vi "Get next acquisition state.vi"(10 "Acquisition order":T2(ring), 11 "Acquisition cluster in":T1={"Save path"=path "D:/DATA_2018", "t frame"=0, "bookmark #"=0, "Z-current"=0, "Channel"=0, "total t frames"=0, "Total bookmarks"=0, "Total z steps"=0, "Total channels"=0, "Gain 1"=100, "Gain 2"=100, "Gain 3"=100, "Gain 4"=100, "Exposure 1"=100.0, "Exposure 2"=100.0, "Exposure 3"=100.0, "Exposure 4"=100.0, "Channel 1"="Red", "Channel 2"="None", "Channel 3"="None", "Channel 4"="None", "Bookmarks?"=FALSE, "Acquisition order"=enum."C-T-Z-B", "t-delay"=0.0, "z-step"=1.0, "Total Images"=1, "Start position"=[], "Piezo radio"=enum."Piezo off", "Piezo Step X"=20.0, "Piezo Step Y"=20.0, "Piezo Step Z"=20.0, "Piezo X current"=0.0, "Piezo Y current"=0.0, "Piezo Z current"=0.0, "LED illumination"=TRUE, "Piezo Amp X"=0.0, "Piezo Amp Y"=0.0, "Piezo Amp Z"=0.0}) -> (0 "Next state":T3 caption="States", 3 "Acquisition cluster out":T1={"Save path"=path "D:/DATA_2018", "t frame"=0, "bookmark #"=0, "Z-current"=0, "Channel"=0, "total t frames"=0, "Total bookmarks"=0, "Total z steps"=0, "Total channels"=0, "Gain 1"=100, "Gain 2"=100, "Gain 3"=100, "Gain 4"=100, "Exposure 1"=100.0, "Exposure 2"=100.0, "Exposure 3"=100.0, "Exposure 4"=100.0, "Channel 1"="Red", "Channel 2"="None", "Channel 3"="None", "Channel 4"="None", "Bookmarks?"=FALSE, "Acquisition order"=enum."C-T-Z-B", "t-delay"=0.0, "z-step"=1.0, "Total Images"=1, "Start position"=[], "Piezo radio"=enum."Piezo off", "Piezo Step X"=20.0, "Piezo Step Y"=20.0, "Piezo Step Z"=20.0, "Piezo X current"=0.0, "Piezo Y current"=0.0, "Piezo Z current"=0.0, "LED illumination"=TRUE, "Piezo Amp X"=0.0, "Piezo Amp Y"=0.0, "Piezo Amp Z"=0.0})   [LabVIEW 2017]
uses:
  <instrlib>/TLDC4100/TLDC4100.llb/z_StateMachineVorlage.ctl
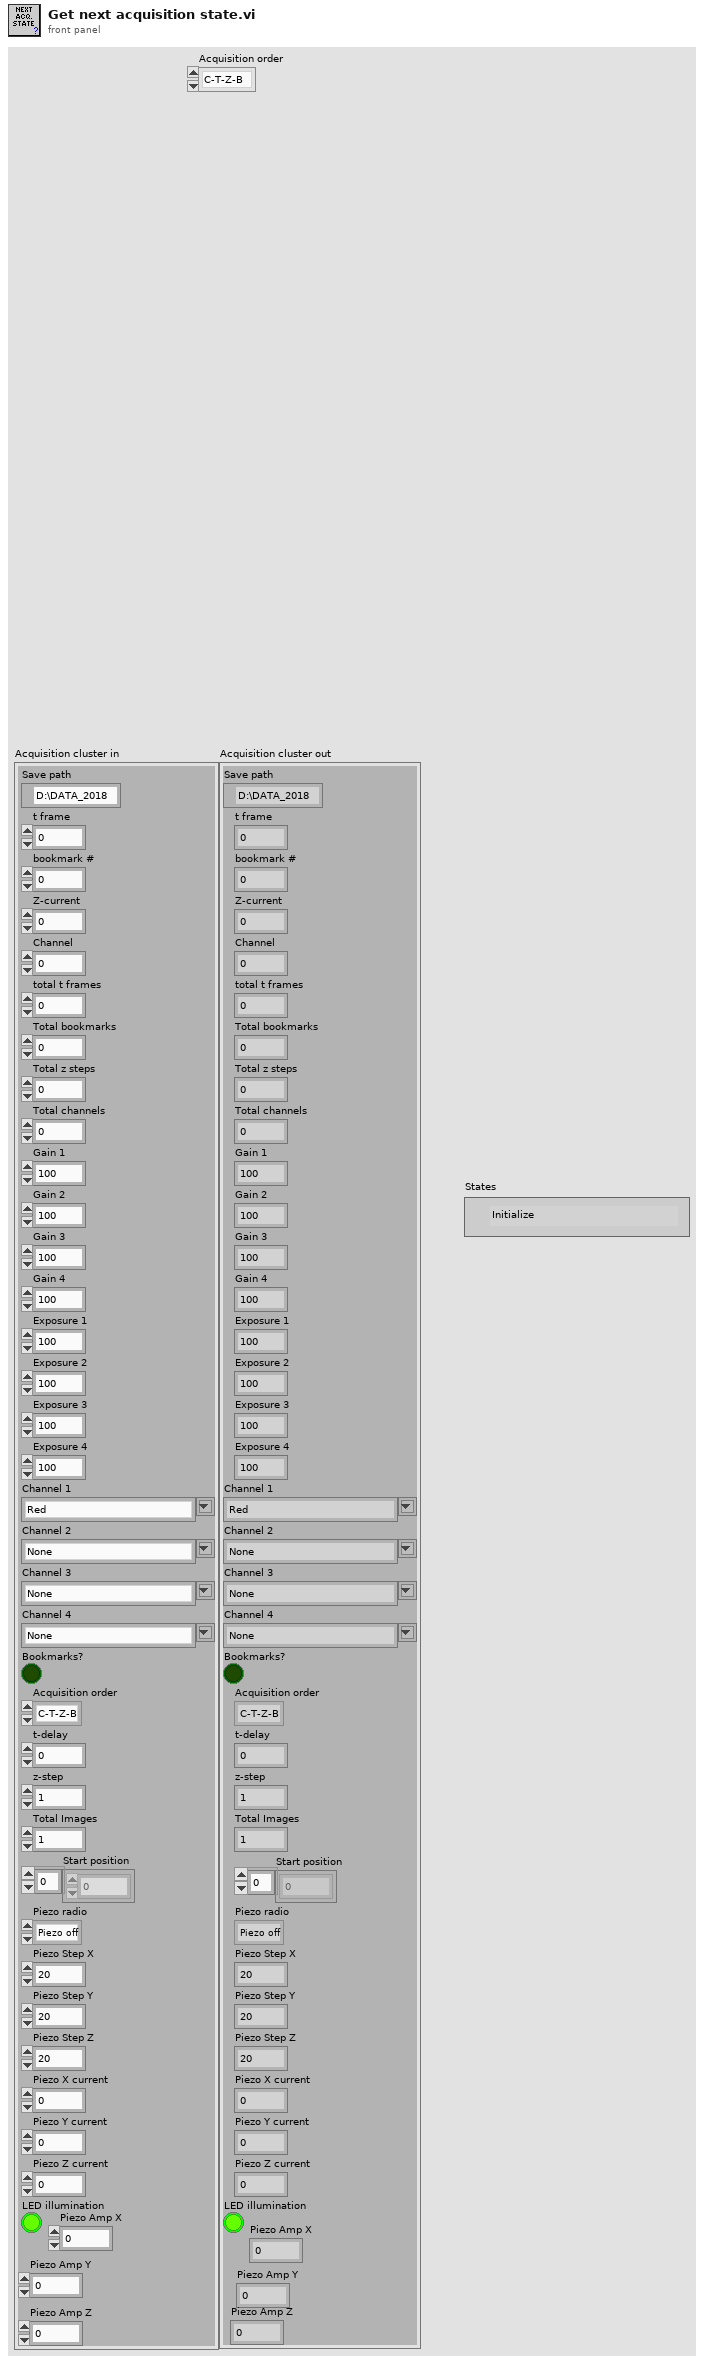
[diagram p1: front panel]
types:
  T1 = cluster{"Save path":path, "t frame":i32, "bookmark #":i32, "Z-current":i32, "Channel":i32, "total t frames":i32, "Total bookmarks":i32, "Total z steps":i32, "Total channels":i32, "Gain 1":i32, "Gain 2":i32, "Gain 3":i32, "Gain 4":i32, "Exposure 1":dbl, "Exposure 2":dbl, "Exposure 3":dbl, "Exposure 4":dbl, "Channel 1":string, "Channel 2":string, "Channel 3":string, "Channel 4":string, "Bookmarks?":bool, "Acquisition order":enum16{"C-T-Z-B", "C-T-B-Z", "C-Z-T-B", "C-Z-B-T", "C-B-T-Z", "C-B-Z-T", "T-C-Z-B", "T-C-B-Z", "T-Z-C-B", "T-Z-B-C", "T-B-C-Z", "T-B-Z-C", "Z-C-T-B", "Z-C-B-T", "Z-T-C-B", "Z-T-B-C", "Z-B-C-T", "Z-B-T-C", "B-C-T-Z", "B-C-Z-T", "B-Z-C-T", "B-Z-T-C", "B-T-C-Z", "B-T-Z-C"}, "t-delay":dbl, "z-step":dbl, "Total Images":i32, "Start position":dbl[], "Piezo radio":enum32{"Piezo off", "Piezo wiggle", "Piezo step"}, "Piezo Step X":dbl, "Piezo Step Y":dbl, "Piezo Step Z":dbl, "Piezo X current":dbl, "Piezo Y current":dbl, "Piezo Z current":dbl, "LED illumination":bool, "Piezo Amp X":dbl, "Piezo Amp Y":dbl, "Piezo Amp Z":dbl}
  T2 = enum16{"C-T-Z-B", "C-T-B-Z", "C-Z-T-B", "C-Z-B-T", "C-B-T-Z", "C-B-Z-T", "T-C-Z-B", "T-C-B-Z", "T-Z-C-B", "T-Z-B-C", "T-B-C-Z", "T-B-Z-C", "Z-C-T-B", "Z-C-B-T", "Z-T-C-B", "Z-T-B-C", "Z-B-C-T", "Z-B-T-C", "B-C-T-Z", "B-C-Z-T", "B-Z-C-T", "B-Z-T-C", "B-T-C-Z", "B-T-Z-C"}
  T3 = typedef "z_StateMachineVorlage.ctl" = enum16{"Initialize", "1", "2", "3", "4", "5", "6", "7", "8", "9", "10", "11", "12", "13", "14", "15", "20", "25", "30", "35", "40", "45", "50", "55", "59", "60", "65", "70", "75", "76", "77", "78", "79", "80", "85", "90", "91", "92", "93", "94", "95", "96", "97", "98", "99", "100", "105", "110", "120", "130", "140", "150", "160", "170", "180", "190", "200", "201", "202", "203", "205", "210", "215", "220", "230", "240", "245", "250", "255", "260", "270", "280", "290", "300", "310", "313", "315", "318", "320", "330", "340", "350", "360", "370", "380", "390", "400", "410", "420", "430", "440", "450", "460", "470", "480", "490", "500", "501", "502", "503", "504", "505", "506", "507", "510", "511", "512", "513", "514", "520", "523", "525", "528", "530", "540", "550", "560", "570", "580", "590", "591", "592", "593", "600", "601", "602", "605", "610", "620", "630", "640", "650", "660", "670", "680", "690", "700", "710", "720", "730", "740", "750", "760", "770", "780", "790", "800", "810", "820", "830", "840", "850", "860", "870", "880", "890", "900", "910", "920", "930", "940", "950", "960", "970", "980", "990", "1000", "1010", "1020", "1030", "1040", "1050", "1060", "1070", "1080", "1090", "1100", "1110", "1120", "1130", "1140", "1150", "1160", "1170", "1180", "1190", "1200", "1210", "1220", "1230", "1240", "1250", "1260", "1270", "1280", "1290", "1300", "1310", "1320", "1330", "1340", "1350", "1360", "1370", "1380", "1390", "1400", "1410", "1420", "1430", "1440", "1450", "1460", "1470", "1480", "1490", "1500", "Fehler I", "Fehler II", "Fehler III", "Fehler IV", "Fehler V", "Fehler VI", "Fehler VII", "Fehler VIII", "Fehler IX", "Fehler X", "Stop"}
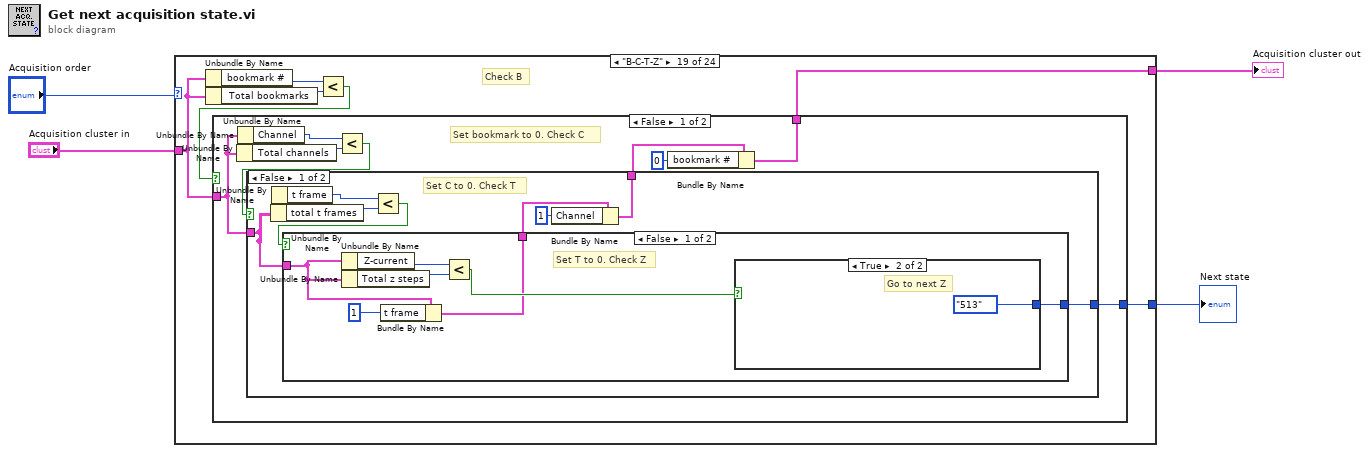
[diagram p0: block diagram]
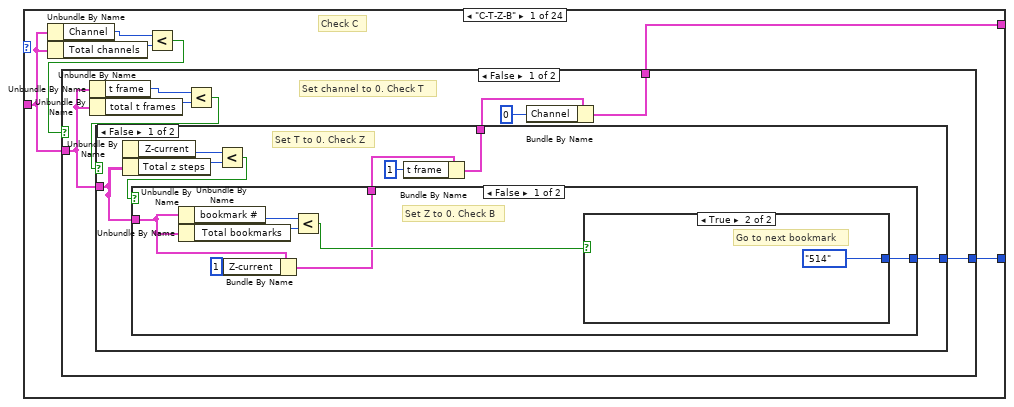
[diagram p2: hidden frame]
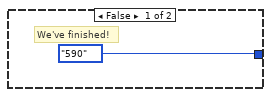
[diagram p3: hidden frame]
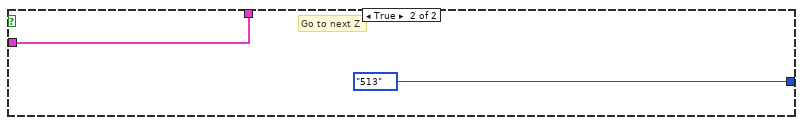
[diagram p4: hidden frame]
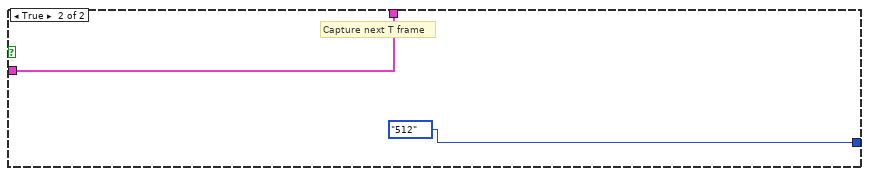
[diagram p5: hidden frame]
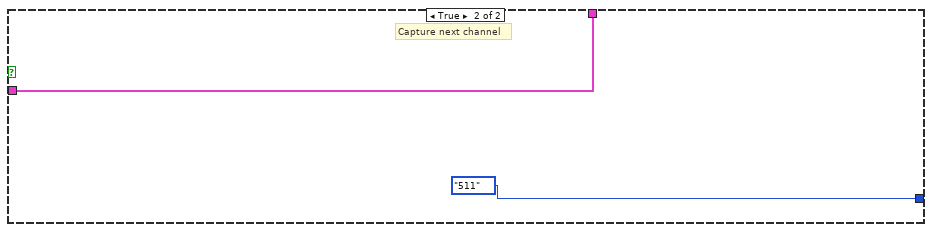
[diagram p6: hidden frame]
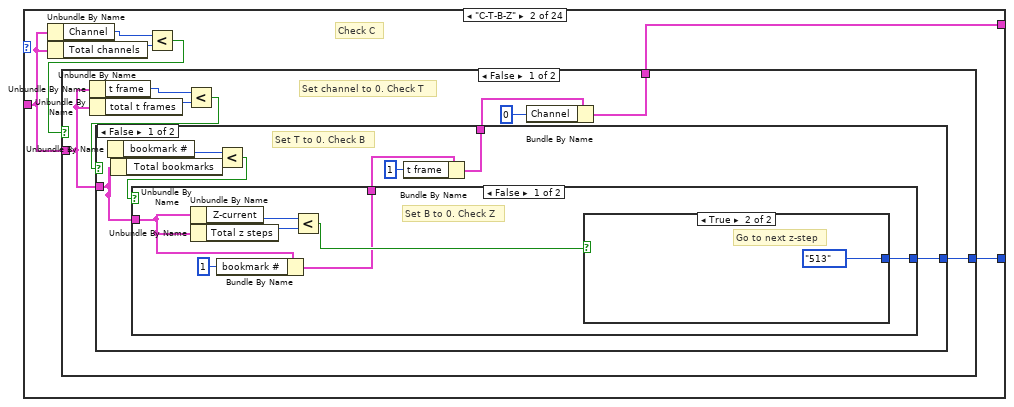
[diagram p7: hidden frame]
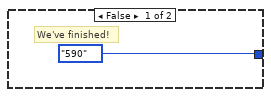
[diagram p8: hidden frame]
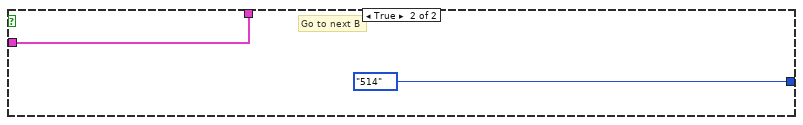
[diagram p9: hidden frame]
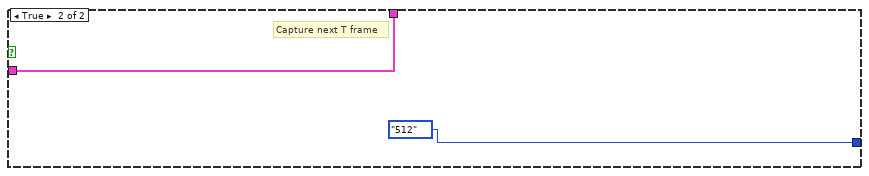
[diagram p10: hidden frame]
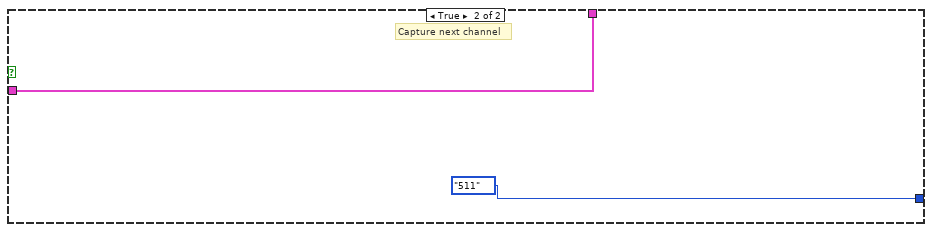
[diagram p11: hidden frame]
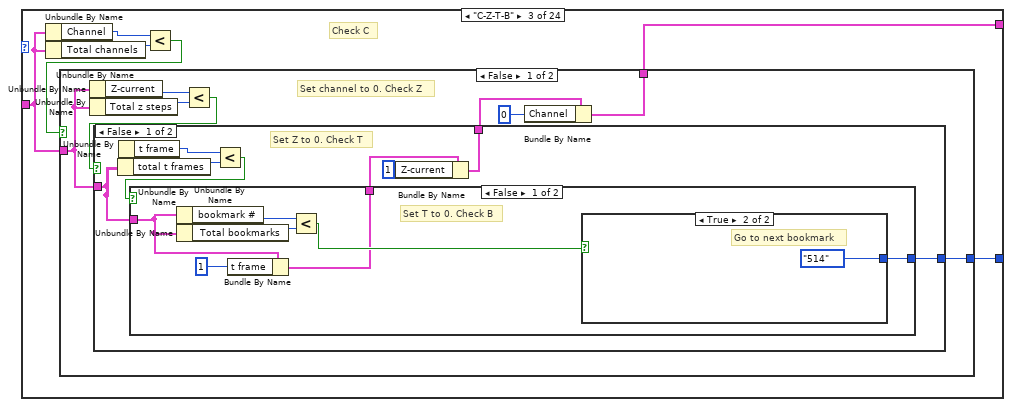
[diagram p12: hidden frame]
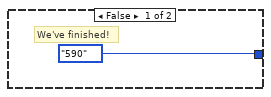
[diagram p13: hidden frame]
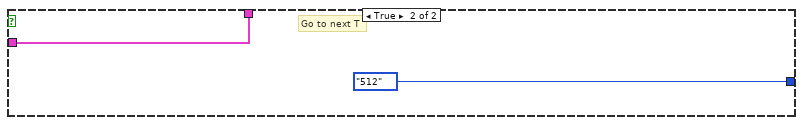
[diagram p14: hidden frame]
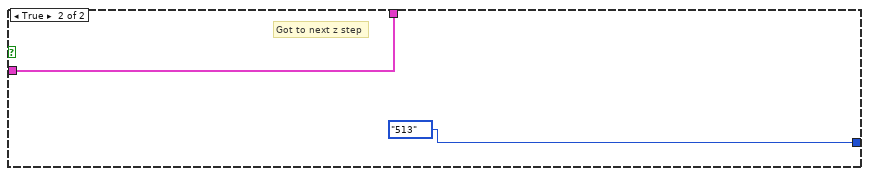
[diagram p15: hidden frame]
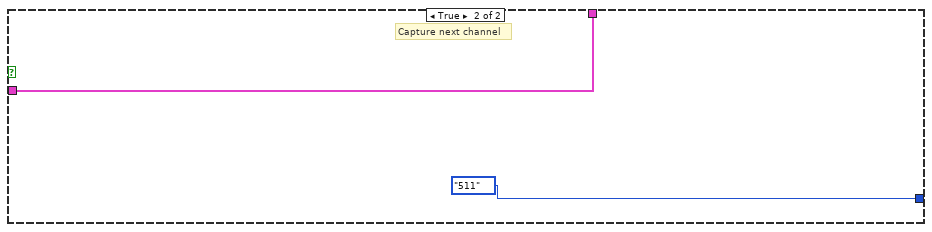
[diagram p16: hidden frame]
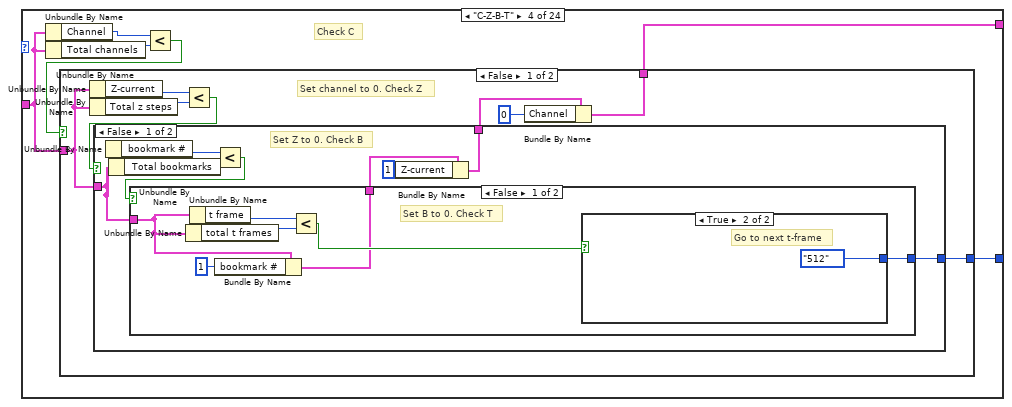
[diagram p17: hidden frame]
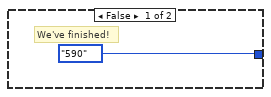
[diagram p18: hidden frame]
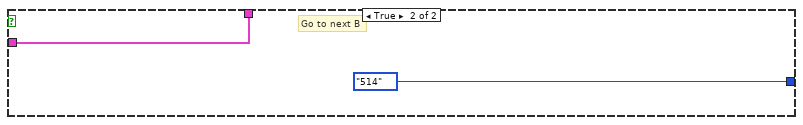
[diagram p19: hidden frame]
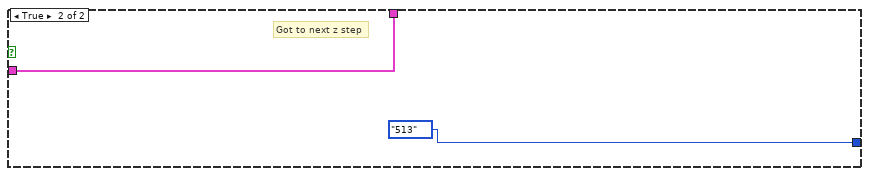
[diagram p20: hidden frame]
diagram:
  n1 = case shown="\"B-C-T-Z\"" "Acquisition order" {
    tunnel: "Acquisition cluster in" -> [w7 w44 w81 w118 w155 w192 w229 w266 w303 w340 w377 w414 w451 w488 w525 w562 w599 w636 w673 w710 w747 w784 w821 w858]
    tunnel: [w6 w43 w80 w117 w154 w191 w228 w265 w302 w339 w376 w413 w450 w487 w524 w561 w598 w635 w672 w709 w746 w783 w820 w857] -> w3
    tunnel: [w5 w42 w79 w116 w153 w190 w227 w264 w301 w338 w375 w412 w449 w486 w523 w560 w597 w634 w671 w708 w745 w782 w819 w856] -> w1
    frame "C-T-Z-B" {
      # "Check C"
      n2 = Unbundle By Name(w7) -> ("Channel"=w10:i32)
      n3 = Unbundle By Name(w7) -> ("Total channels"=w9:i32)
      n4 = Less?(x=w10, y=w9) -> (x < y?=w8:bool)
      n5 = case shown="False" w8 {
        tunnel: w7 -> [w14 w40]
        tunnel: [w15 z_StateMachineVorlage."511" ("States")] -> w6
        tunnel: [w11 w40] -> w5
        frame False {
          # "Set channel to 0. Check T"
          n6 = Unbundle By Name(w14) -> ("t frame"=w17:i32)
          n7 = Unbundle By Name(w14) -> ("total t frames"=w18:i32)
          n8 = Less?(x=w17, y=w18) -> (x < y?=w16:bool)
          n9 = case shown="False" w16 {
            tunnel: [w23 z_StateMachineVorlage."512" ("States")] -> w15
            tunnel: w14 -> [w22 w38]
            tunnel: [w19 w38] -> w12
            frame False {
              # "Set T to 0. Check Z"
              n10 = Unbundle By Name(w22) -> ("Z-current"=w26:i32)
              n11 = Unbundle By Name(w22) -> ("Total z steps"=w25:i32)
              n12 = Less?(x=w26, y=w25) -> (x < y?=w24:bool)
              n13 = case shown="False" w24 {
                tunnel: w22 -> [w29 w36]
                tunnel: [w30 z_StateMachineVorlage."513" ("States")] -> w23
                tunnel: [w27 w36] -> w20
                frame False {
                  # "Set Z to 0. Check B"
                  n14 = Unbundle By Name(w29) -> ("bookmark #"=w32:i32)
                  n15 = Unbundle By Name(w29) -> ("Total bookmarks"=w33:i32)
                  n16 = Bundle By Name(cluster=w29, "Z-current"=1 ("Z-step")) -> (w27:T1)
                  n17 = Less?(x=w32, y=w33) -> (x < y?=w31:bool)
                  n18 = case shown="True" w31 {
                    tunnel: [z_StateMachineVorlage."590" ("States") z_StateMachineVorlage."514" ("States")] -> w30
                    frame False {
                      # "We've finished!"
                    }
                    frame True {
                      # "Go to next bookmark"
                    }
                  }
                }
                frame True {
                  # "Go to next Z"
                }
              }
              n19 = Bundle By Name(cluster=w20, "t frame"=1 ("Z-step")) -> (w19:T1)
            }
            frame True {
              # "Capture next T frame"
            }
          }
          n20 = Bundle By Name(cluster=w12, "Channel"=0 ("Z-step")) -> (w11:T1)
        }
        frame True {
          # "Capture next channel"
        }
      }
    }
    frame "C-T-B-Z" {
      # "Check C"
      n21 = Unbundle By Name(w44) -> ("Channel"=w47:i32)
      n22 = Unbundle By Name(w44) -> ("Total channels"=w46:i32)
      n23 = Less?(x=w47, y=w46) -> (x < y?=w45:bool)
      n24 = case shown="False" w45 {
        tunnel: w44 -> [w51 w77]
        tunnel: [w52 z_StateMachineVorlage."511" ("States")] -> w43
        tunnel: [w48 w77] -> w42
        frame False {
          # "Set channel to 0. Check T"
          n25 = Unbundle By Name(w51) -> ("t frame"=w54:i32)
          n26 = Unbundle By Name(w51) -> ("total t frames"=w55:i32)
          n27 = Less?(x=w54, y=w55) -> (x < y?=w53:bool)
          n28 = case shown="False" w53 {
            tunnel: [w60 z_StateMachineVorlage."512" ("States")] -> w52
            tunnel: w51 -> [w59 w75]
            tunnel: [w56 w75] -> w49
            frame False {
              # "Set T to 0. Check B"
              n29 = Unbundle By Name(w59) -> ("bookmark #"=w63:i32)
              n30 = Unbundle By Name(w59) -> ("Total bookmarks"=w62:i32)
              n31 = Less?(x=w63, y=w62) -> (x < y?=w61:bool)
              n32 = case shown="False" w61 {
                tunnel: w59 -> [w66 w73]
                tunnel: [w67 z_StateMachineVorlage."514" ("States")] -> w60
                tunnel: [w64 w73] -> w57
                frame False {
                  # "Set B to 0. Check Z"
                  n33 = Unbundle By Name(w66) -> ("Z-current"=w69:i32)
                  n34 = Unbundle By Name(w66) -> ("Total z steps"=w70:i32)
                  n35 = Bundle By Name(cluster=w66, "bookmark #"=1 ("Z-step")) -> (w64:T1)
                  n36 = Less?(x=w69, y=w70) -> (x < y?=w68:bool)
                  n37 = case shown="True" w68 {
                    tunnel: [z_StateMachineVorlage."590" ("States") z_StateMachineVorlage."513" ("States")] -> w67
                    frame False {
                      # "We've finished!"
                    }
                    frame True {
                      # "Go to next z-step"
                    }
                  }
                }
                frame True {
                  # "Go to next B"
                }
              }
              n38 = Bundle By Name(cluster=w57, "t frame"=1 ("Z-step")) -> (w56:T1)
            }
            frame True {
              # "Capture next T frame"
            }
          }
          n39 = Bundle By Name(cluster=w49, "Channel"=0 ("Z-step")) -> (w48:T1)
        }
        frame True {
          # "Capture next channel"
        }
      }
    }
    frame "C-Z-T-B" {
      # "Check C"
      n40 = Unbundle By Name(w81) -> ("Channel"=w84:i32)
      n41 = Unbundle By Name(w81) -> ("Total channels"=w83:i32)
      n42 = Less?(x=w84, y=w83) -> (x < y?=w82:bool)
      n43 = case shown="False" w82 {
        tunnel: w81 -> [w88 w114]
        tunnel: [w89 z_StateMachineVorlage."511" ("States")] -> w80
        tunnel: [w85 w114] -> w79
        frame False {
          # "Set channel to 0. Check Z"
          n44 = Unbundle By Name(w88) -> ("Z-current"=w91:i32)
          n45 = Unbundle By Name(w88) -> ("Total z steps"=w92:i32)
          n46 = Less?(x=w91, y=w92) -> (x < y?=w90:bool)
          n47 = case shown="False" w90 {
            tunnel: [w97 z_StateMachineVorlage."513" ("States")] -> w89
            tunnel: w88 -> [w96 w112]
            tunnel: [w93 w112] -> w86
            frame False {
              # "Set Z to 0. Check T"
              n48 = Unbundle By Name(w96) -> ("total t frames"=w99:i32)
              n49 = Unbundle By Name(w96) -> ("t frame"=w100:i32)
              n50 = Less?(x=w100, y=w99) -> (x < y?=w98:bool)
              n51 = case shown="False" w98 {
                tunnel: w96 -> [w103 w110]
                tunnel: [w104 z_StateMachineVorlage."512" ("States")] -> w97
                tunnel: [w101 w110] -> w94
                frame False {
                  # "Set T to 0. Check B"
                  n52 = Unbundle By Name(w103) -> ("bookmark #"=w106:i32)
                  n53 = Unbundle By Name(w103) -> ("Total bookmarks"=w107:i32)
                  n54 = Bundle By Name(cluster=w103, "t frame"=1 ("Z-step")) -> (w101:T1)
                  n55 = Less?(x=w106, y=w107) -> (x < y?=w105:bool)
                  n56 = case shown="True" w105 {
                    tunnel: [z_StateMachineVorlage."590" ("States") z_StateMachineVorlage."514" ("States")] -> w104
                    frame False {
                      # "We've finished!"
                    }
                    frame True {
                      # "Go to next bookmark"
                    }
                  }
                }
                frame True {
                  # "Go to next T"
                }
              }
              n57 = Bundle By Name(cluster=w94, "Z-current"=1 ("Z-step")) -> (w93:T1)
            }
            frame True {
              # "Got to next z step"
            }
          }
          n58 = Bundle By Name(cluster=w86, "Channel"=0 ("Z-step")) -> (w85:T1)
        }
        frame True {
          # "Capture next channel"
        }
      }
    }
    frame "C-Z-B-T" {
      # "Check C"
      n59 = Unbundle By Name(w118) -> ("Channel"=w121:i32)
      n60 = Unbundle By Name(w118) -> ("Total channels"=w120:i32)
      n61 = Less?(x=w121, y=w120) -> (x < y?=w119:bool)
      n62 = case shown="False" w119 {
        tunnel: w118 -> [w125 w151]
        tunnel: [w126 z_StateMachineVorlage."511" ("States")] -> w117
        tunnel: [w122 w151] -> w116
        frame False {
          # "Set channel to 0. Check Z"
          n63 = Unbundle By Name(w125) -> ("Z-current"=w128:i32)
          n64 = Unbundle By Name(w125) -> ("Total z steps"=w129:i32)
          n65 = Less?(x=w128, y=w129) -> (x < y?=w127:bool)
          n66 = case shown="False" w127 {
            tunnel: [w134 z_StateMachineVorlage."513" ("States")] -> w126
            tunnel: w125 -> [w133 w149]
            tunnel: [w130 w149] -> w123
            frame False {
              # "Set Z to 0. Check B"
              n67 = Unbundle By Name(w133) -> ("bookmark #"=w137:i32)
              n68 = Unbundle By Name(w133) -> ("Total bookmarks"=w136:i32)
              n69 = Less?(x=w137, y=w136) -> (x < y?=w135:bool)
              n70 = case shown="False" w135 {
                tunnel: w133 -> [w140 w147]
                tunnel: [w141 z_StateMachineVorlage."514" ("States")] -> w134
                tunnel: [w138 w147] -> w131
                frame False {
                  # "Set B to 0. Check T"
                  n71 = Unbundle By Name(w140) -> ("total t frames"=w144:i32)
                  n72 = Unbundle By Name(w140) -> ("t frame"=w143:i32)
                  n73 = Bundle By Name(cluster=w140, "bookmark #"=1 ("Z-step")) -> (w138:T1)
                  n74 = Less?(x=w143, y=w144) -> (x < y?=w142:bool)
                  n75 = case shown="True" w142 {
                    tunnel: [z_StateMachineVorlage."590" ("States") z_StateMachineVorlage."512" ("States")] -> w141
                    frame False {
                      # "We've finished!"
                    }
                    frame True {
                      # "Go to next t-frame"
                    }
                  }
                }
                frame True {
                  # "Go to next B"
                }
              }
              n76 = Bundle By Name(cluster=w131, "Z-current"=1 ("Z-step")) -> (w130:T1)
            }
            frame True {
              # "Got to next z step"
            }
          }
          n77 = Bundle By Name(cluster=w123, "Channel"=0 ("Z-step")) -> (w122:T1)
        }
        frame True {
          # "Capture next channel"
        }
      }
    }
    frame "C-B-T-Z" {
      # "Check C"
      n78 = Unbundle By Name(w155) -> ("Channel"=w158:i32)
      n79 = Unbundle By Name(w155) -> ("Total channels"=w157:i32)
      n80 = Less?(x=w158, y=w157) -> (x < y?=w156:bool)
      n81 = case shown="False" w156 {
        tunnel: w155 -> [w162 w188]
        tunnel: [w163 z_StateMachineVorlage."511" ("States")] -> w154
        tunnel: [w159 w188] -> w153
        frame False {
          # "Set channel to 0. Check Z"
          n82 = Unbundle By Name(w162) -> ("bookmark #"=w165:i32)
          n83 = Unbundle By Name(w162) -> ("Total bookmarks"=w166:i32)
          n84 = Less?(x=w165, y=w166) -> (x < y?=w164:bool)
          n85 = case shown="False" w164 {
            tunnel: [w171 z_StateMachineVorlage."514" ("States")] -> w163
            tunnel: w162 -> [w170 w186]
            tunnel: [w167 w186] -> w160
            frame False {
              # "Set B to 0. Check T"
              n86 = Unbundle By Name(w170) -> ("total t frames"=w173:i32)
              n87 = Unbundle By Name(w170) -> ("t frame"=w174:i32)
              n88 = Less?(x=w174, y=w173) -> (x < y?=w172:bool)
              n89 = case shown="False" w172 {
                tunnel: w170 -> [w177 w184]
                tunnel: [w178 z_StateMachineVorlage."512" ("States")] -> w171
                tunnel: [w175 w184] -> w168
                frame False {
                  # "Set T to 0. Check Z"
                  n90 = Unbundle By Name(w177) -> ("Z-current"=w180:i32)
                  n91 = Unbundle By Name(w177) -> ("Total z steps"=w181:i32)
                  n92 = Bundle By Name(cluster=w177, "t frame"=1 ("Z-step")) -> (w175:T1)
                  n93 = Less?(x=w180, y=w181) -> (x < y?=w179:bool)
                  n94 = case shown="True" w179 {
                    tunnel: [z_StateMachineVorlage."590" ("States") z_StateMachineVorlage."513" ("States")] -> w178
                    frame False {
                      # "We've finished!"
                    }
                    frame True {
                      # "Go to next z-step"
                    }
                  }
                }
                frame True {
                  # "Go to next T"
                }
              }
              n95 = Bundle By Name(cluster=w168, "bookmark #"=1 ("Z-step")) -> (w167:T1)
            }
            frame True {
              # "Got to next bookmark"
            }
          }
          n96 = Bundle By Name(cluster=w160, "Channel"=0 ("Z-step")) -> (w159:T1)
        }
        frame True {
          # "Capture next channel"
        }
      }
    }
    frame "C-B-Z-T" {
      # "Check C"
      n97 = Unbundle By Name(w192) -> ("Channel"=w195:i32)
      n98 = Unbundle By Name(w192) -> ("Total channels"=w194:i32)
      n99 = Less?(x=w195, y=w194) -> (x < y?=w193:bool)
      n100 = case shown="False" w193 {
        tunnel: w192 -> [w199 w225]
        tunnel: [w200 z_StateMachineVorlage."511" ("States")] -> w191
        tunnel: [w196 w225] -> w190
        frame False {
          # "Set channel to 0. Check Z"
          n101 = Unbundle By Name(w199) -> ("bookmark #"=w202:i32)
          n102 = Unbundle By Name(w199) -> ("Total bookmarks"=w203:i32)
          n103 = Less?(x=w202, y=w203) -> (x < y?=w201:bool)
          n104 = case shown="False" w201 {
            tunnel: [w208 z_StateMachineVorlage."514" ("States")] -> w200
            tunnel: w199 -> [w207 w223]
            tunnel: [w204 w223] -> w197
            frame False {
              # "Set B to 0. Check Z"
              n105 = Unbundle By Name(w207) -> ("Z-current"=w211:i32)
              n106 = Unbundle By Name(w207) -> ("Total z steps"=w210:i32)
              n107 = Less?(x=w211, y=w210) -> (x < y?=w209:bool)
              n108 = case shown="False" w209 {
                tunnel: w207 -> [w214 w221]
                tunnel: [w215 z_StateMachineVorlage."513" ("States")] -> w208
                tunnel: [w212 w221] -> w205
                frame False {
                  # "Set Z to 0. Check T"
                  n109 = Unbundle By Name(w214) -> ("total t frames"=w218:i32)
                  n110 = Unbundle By Name(w214) -> ("t frame"=w217:i32)
                  n111 = Bundle By Name(cluster=w214, "Z-current"=1 ("Z-step")) -> (w212:T1)
                  n112 = Less?(x=w217, y=w218) -> (x < y?=w216:bool)
                  n113 = case shown="True" w216 {
                    tunnel: [z_StateMachineVorlage."590" ("States") z_StateMachineVorlage."512" ("States")] -> w215
                    frame False {
                      # "We've finished!"
                    }
                    frame True {
                      # "Go to next t-frame"
                    }
                  }
                }
                frame True {
                  # "Go to next Z"
                }
              }
              n114 = Bundle By Name(cluster=w205, "bookmark #"=1 ("Z-step")) -> (w204:T1)
            }
            frame True {
              # "Got to next bookmark"
            }
          }
          n115 = Bundle By Name(cluster=w197, "Channel"=0 ("Z-step")) -> (w196:T1)
        }
        frame True {
          # "Capture next channel"
        }
      }
    }
    frame "T-C-Z-B" {
      # "Check T"
      n116 = Unbundle By Name(w229) -> ("t frame"=w232:i32)
      n117 = Unbundle By Name(w229) -> ("total t frames"=w231:i32)
      n118 = Less?(x=w232, y=w231) -> (x < y?=w230:bool)
      n119 = case shown="False" w230 {
        tunnel: w229 -> [w236 w262]
        tunnel: [w237 z_StateMachineVorlage."512" ("States")] -> w228
        tunnel: [w233 w262] -> w227
        frame False {
          # "Set t-frame to 0. Check C"
          n120 = Unbundle By Name(w236) -> ("Channel"=w239:i32)
          n121 = Unbundle By Name(w236) -> ("Total channels"=w240:i32)
          n122 = Less?(x=w239, y=w240) -> (x < y?=w238:bool)
          n123 = case shown="False" w238 {
            tunnel: [w245 z_StateMachineVorlage."511" ("States")] -> w237
            tunnel: w236 -> [w244 w260]
            tunnel: [w241 w260] -> w234
            frame False {
              # "Set C to 0. Check Z"
              n124 = Unbundle By Name(w244) -> ("Z-current"=w248:i32)
              n125 = Unbundle By Name(w244) -> ("Total z steps"=w247:i32)
              n126 = Less?(x=w248, y=w247) -> (x < y?=w246:bool)
              n127 = case shown="False" w246 {
                tunnel: w244 -> [w251 w258]
                tunnel: [w252 z_StateMachineVorlage."513" ("States")] -> w245
                tunnel: [w249 w258] -> w242
                frame False {
                  # "Set Z to 0. Check B"
                  n128 = Unbundle By Name(w251) -> ("bookmark #"=w254:i32)
                  n129 = Unbundle By Name(w251) -> ("Total bookmarks"=w255:i32)
                  n130 = Bundle By Name(cluster=w251, "Z-current"=1 ("Z-step")) -> (w249:T1)
                  n131 = Less?(x=w254, y=w255) -> (x < y?=w253:bool)
                  n132 = case shown="True" w253 {
                    tunnel: [z_StateMachineVorlage."590" ("States") z_StateMachineVorlage."514" ("States")] -> w252
                    frame False {
                      # "We've finished!"
                    }
                    frame True {
                      # "Go to next bookmark"
                    }
                  }
                }
                frame True {
                  # "Go to next Z"
                }
              }
              n133 = Bundle By Name(cluster=w242, "Channel"=1 ("Z-step")) -> (w241:T1)
            }
            frame True {
              # "Capture next channel"
            }
          }
          n134 = Bundle By Name(cluster=w234, "t frame"=0 ("Z-step")) -> (w233:T1)
        }
        frame True {
          # "Capture next t-frame"
        }
      }
    }
    frame "T-C-B-Z" {
      # "Check T"
      n135 = Unbundle By Name(w266) -> ("t frame"=w269:i32)
      n136 = Unbundle By Name(w266) -> ("total t frames"=w268:i32)
      n137 = Less?(x=w269, y=w268) -> (x < y?=w267:bool)
      n138 = case shown="False" w267 {
        tunnel: w266 -> [w271 w299]
        tunnel: [w270 z_StateMachineVorlage."512" ("States")] -> w265
        tunnel: [w274 w299] -> w264
        frame False {
          # "Set t-frame to 0. Check C"
          n139 = Unbundle By Name(w271) -> ("Channel"=w276:i32)
          n140 = Unbundle By Name(w271) -> ("Total channels"=w277:i32)
          n141 = Less?(x=w276, y=w277) -> (x < y?=w272:bool)
          n142 = case shown="False" w272 {
            tunnel: [w282 z_StateMachineVorlage."511" ("States")] -> w270
            tunnel: w271 -> [w281 w297]
            tunnel: [w278 w297] -> w273
            frame False {
              # "Set C to 0. Check B"
              n143 = Unbundle By Name(w281) -> ("bookmark #"=w285:i32)
              n144 = Unbundle By Name(w281) -> ("Total bookmarks"=w284:i32)
              n145 = Less?(x=w285, y=w284) -> (x < y?=w283:bool)
              n146 = case shown="False" w283 {
                tunnel: w281 -> [w288 w295]
                tunnel: [w289 z_StateMachineVorlage."514" ("States")] -> w282
                tunnel: [w286 w295] -> w279
                frame False {
                  # "Set B to 0. Check Z"
                  n147 = Unbundle By Name(w288) -> ("Z-current"=w291:i32)
                  n148 = Unbundle By Name(w288) -> ("Total z steps"=w292:i32)
                  n149 = Bundle By Name(cluster=w288, "bookmark #"=1 ("Z-step")) -> (w286:T1)
                  n150 = Less?(x=w291, y=w292) -> (x < y?=w290:bool)
                  n151 = case shown="True" w290 {
                    tunnel: [z_StateMachineVorlage."590" ("States") z_StateMachineVorlage."513" ("States")] -> w289
                    frame False {
                      # "We've finished!"
                    }
                    frame True {
                      # "Go to next z-step"
                    }
                  }
                }
                frame True {
                  # "Go to next B"
                }
              }
              n152 = Bundle By Name(cluster=w279, "Channel"=1 ("Z-step")) -> (w278:T1)
            }
            frame True {
              # "Capture next channel"
            }
          }
          n153 = Bundle By Name(cluster=w273, "t frame"=0 ("Z-step")) -> (w274:T1)
        }
        frame True {
          # "Capture next t-frame"
        }
      }
    }
    frame "T-Z-C-B" {
      # "Check T"
      n154 = Unbundle By Name(w303) -> ("t frame"=w306:i32)
      n155 = Unbundle By Name(w303) -> ("total t frames"=w305:i32)
      n156 = Less?(x=w306, y=w305) -> (x < y?=w304:bool)
      n157 = case shown="False" w304 {
        tunnel: w303 -> [w308 w336]
        tunnel: [w307 z_StateMachineVorlage."512" ("States")] -> w302
        tunnel: [w311 w336] -> w301
        frame False {
          # "Set t-frame to 0. Check Z"
          n158 = Unbundle By Name(w308) -> ("Z-current"=w313:i32)
          n159 = Unbundle By Name(w308) -> ("Total z steps"=w314:i32)
          n160 = Less?(x=w313, y=w314) -> (x < y?=w309:bool)
          n161 = case shown="False" w309 {
            tunnel: [w319 z_StateMachineVorlage."513" ("States")] -> w307
            tunnel: w308 -> [w318 w334]
            tunnel: [w315 w334] -> w310
            frame False {
              # "Set Z to 0. Check C"
              n162 = Unbundle By Name(w318) -> ("Total channels"=w321:i32)
              n163 = Unbundle By Name(w318) -> ("Channel"=w322:i32)
              n164 = Less?(x=w322, y=w321) -> (x < y?=w320:bool)
              n165 = case shown="False" w320 {
                tunnel: w318 -> [w325 w332]
                tunnel: [w326 z_StateMachineVorlage."511" ("States")] -> w319
                tunnel: [w323 w332] -> w316
                frame False {
                  # "Set C to 0. Check B"
                  n166 = Unbundle By Name(w325) -> ("bookmark #"=w328:i32)
                  n167 = Unbundle By Name(w325) -> ("Total bookmarks"=w329:i32)
                  n168 = Bundle By Name(cluster=w325, "Channel"=1 ("Z-step")) -> (w323:T1)
                  n169 = Less?(x=w328, y=w329) -> (x < y?=w327:bool)
                  n170 = case shown="True" w327 {
                    tunnel: [z_StateMachineVorlage."590" ("States") z_StateMachineVorlage."514" ("States")] -> w326
                    frame False {
                      # "We've finished!"
                    }
                    frame True {
                      # "Go to next bookmark"
                    }
                  }
                }
                frame True {
                  # "Capture next channel"
                }
              }
              n171 = Bundle By Name(cluster=w316, "Z-current"=1 ("Z-step")) -> (w315:T1)
            }
            frame True {
              # "Go to next Z step"
            }
          }
          n172 = Bundle By Name(cluster=w310, "t frame"=0 ("Z-step")) -> (w311:T1)
        }
        frame True {
          # "Capture next t-frame"
        }
      }
    }
    frame "T-Z-B-C" {
      # "Check T"
      n173 = Unbundle By Name(w340) -> ("t frame"=w343:i32)
      n174 = Unbundle By Name(w340) -> ("total t frames"=w342:i32)
      n175 = Less?(x=w343, y=w342) -> (x < y?=w341:bool)
      n176 = case shown="False" w341 {
        tunnel: w340 -> [w345 w373]
        tunnel: [w344 z_StateMachineVorlage."512" ("States")] -> w339
        tunnel: [w348 w373] -> w338
        frame False {
          # "Set t-frame to 0. Check Z"
          n177 = Unbundle By Name(w345) -> ("Z-current"=w350:i32)
          n178 = Unbundle By Name(w345) -> ("Total z steps"=w351:i32)
          n179 = Less?(x=w350, y=w351) -> (x < y?=w346:bool)
          n180 = case shown="False" w346 {
            tunnel: [w356 z_StateMachineVorlage."513" ("States")] -> w344
            tunnel: w345 -> [w355 w371]
            tunnel: [w352 w371] -> w347
            frame False {
              # "Set Z to 0. Check B"
              n181 = Unbundle By Name(w355) -> ("bookmark #"=w359:i32)
              n182 = Unbundle By Name(w355) -> ("Total bookmarks"=w358:i32)
              n183 = Less?(x=w359, y=w358) -> (x < y?=w357:bool)
              n184 = case shown="False" w357 {
                tunnel: w355 -> [w362 w369]
                tunnel: [w363 z_StateMachineVorlage."514" ("States")] -> w356
                tunnel: [w360 w369] -> w353
                frame False {
                  # "Set B to 0. Check C"
                  n185 = Unbundle By Name(w362) -> ("Total channels"=w366:i32)
                  n186 = Unbundle By Name(w362) -> ("Channel"=w365:i32)
                  n187 = Bundle By Name(cluster=w362, "bookmark #"=1 ("Z-step")) -> (w360:T1)
                  n188 = Less?(x=w365, y=w366) -> (x < y?=w364:bool)
                  n189 = case shown="True" w364 {
                    tunnel: [z_StateMachineVorlage."590" ("States") z_StateMachineVorlage."511" ("States")] -> w363
                    frame False {
                      # "We've finished!"
                    }
                    frame True {
                      # "Go to next channel"
                    }
                  }
                }
                frame True {
                  # "Capture next bookmark"
                }
              }
              n190 = Bundle By Name(cluster=w353, "Z-current"=1 ("Z-step")) -> (w352:T1)
            }
            frame True {
              # "Go to next z step"
            }
          }
          n191 = Bundle By Name(cluster=w347, "t frame"=0 ("Z-step")) -> (w348:T1)
        }
        frame True {
          # "Capture next t-frame"
        }
      }
    }
    frame "T-B-C-Z" {
      # "Check T"
      n192 = Unbundle By Name(w377) -> ("t frame"=w380:i32)
      n193 = Unbundle By Name(w377) -> ("total t frames"=w379:i32)
      n194 = Less?(x=w380, y=w379) -> (x < y?=w378:bool)
      n195 = case shown="False" w378 {
        tunnel: w377 -> [w382 w410]
        tunnel: [w381 z_StateMachineVorlage."512" ("States")] -> w376
        tunnel: [w385 w410] -> w375
        frame False {
          # "Set t-frame to 0. Check B"
          n196 = Unbundle By Name(w382) -> ("bookmark #"=w387:i32)
          n197 = Unbundle By Name(w382) -> ("Total bookmarks"=w388:i32)
          n198 = Less?(x=w387, y=w388) -> (x < y?=w383:bool)
          n199 = case shown="False" w383 {
            tunnel: [w393 z_StateMachineVorlage."514" ("States")] -> w381
            tunnel: w382 -> [w392 w408]
            tunnel: [w389 w408] -> w384
            frame False {
              # "Set B to 0. Check C"
              n200 = Unbundle By Name(w392) -> ("Total channels"=w395:i32)
              n201 = Unbundle By Name(w392) -> ("Channel"=w396:i32)
              n202 = Less?(x=w396, y=w395) -> (x < y?=w394:bool)
              n203 = case shown="False" w394 {
                tunnel: w392 -> [w399 w406]
                tunnel: [w400 z_StateMachineVorlage."511" ("States")] -> w393
                tunnel: [w397 w406] -> w390
                frame False {
                  # "Set C to 0. Check Z"
                  n204 = Unbundle By Name(w399) -> ("Z-current"=w402:i32)
                  n205 = Unbundle By Name(w399) -> ("Total z steps"=w403:i32)
                  n206 = Bundle By Name(cluster=w399, "Channel"=1 ("Z-step")) -> (w397:T1)
                  n207 = Less?(x=w402, y=w403) -> (x < y?=w401:bool)
                  n208 = case shown="True" w401 {
                    tunnel: [z_StateMachineVorlage."590" ("States") z_StateMachineVorlage."513" ("States")] -> w400
                    frame False {
                      # "We've finished!"
                    }
                    frame True {
                      # "Go to next Z"
                    }
                  }
                }
                frame True {
                  # "Capture next channel"
                }
              }
              n209 = Bundle By Name(cluster=w390, "bookmark #"=1 ("Z-step")) -> (w389:T1)
            }
            frame True {
              # "Go to next bookmark"
            }
          }
          n210 = Bundle By Name(cluster=w384, "t frame"=0 ("Z-step")) -> (w385:T1)
        }
        frame True {
          # "Capture next t-frame"
        }
      }
    }
    frame "T-B-Z-C" {
      # "Check T"
      n211 = Unbundle By Name(w414) -> ("t frame"=w417:i32)
      n212 = Unbundle By Name(w414) -> ("total t frames"=w416:i32)
      n213 = Less?(x=w417, y=w416) -> (x < y?=w415:bool)
      n214 = case shown="False" w415 {
        tunnel: w414 -> [w419 w447]
        tunnel: [w418 z_StateMachineVorlage."512" ("States")] -> w413
        tunnel: [w422 w447] -> w412
        frame False {
          # "Set t-frame to 0. Check B"
          n215 = Unbundle By Name(w419) -> ("bookmark #"=w424:i32)
          n216 = Unbundle By Name(w419) -> ("Total bookmarks"=w425:i32)
          n217 = Less?(x=w424, y=w425) -> (x < y?=w420:bool)
          n218 = case shown="False" w420 {
            tunnel: [w430 z_StateMachineVorlage."514" ("States")] -> w418
            tunnel: w419 -> [w429 w445]
            tunnel: [w426 w445] -> w421
            frame False {
              # "Set B to 0. Check Z"
              n219 = Unbundle By Name(w429) -> ("Z-current"=w433:i32)
              n220 = Unbundle By Name(w429) -> ("Total z steps"=w432:i32)
              n221 = Less?(x=w433, y=w432) -> (x < y?=w431:bool)
              n222 = case shown="False" w431 {
                tunnel: w429 -> [w436 w443]
                tunnel: [w437 z_StateMachineVorlage."513" ("States")] -> w430
                tunnel: [w434 w443] -> w427
                frame False {
                  # "Set Z to 0. Check C"
                  n223 = Unbundle By Name(w436) -> ("Total channels"=w440:i32)
                  n224 = Unbundle By Name(w436) -> ("Channel"=w439:i32)
                  n225 = Bundle By Name(cluster=w436, "Z-current"=1 ("Z-step")) -> (w434:T1)
                  n226 = Less?(x=w439, y=w440) -> (x < y?=w438:bool)
                  n227 = case shown="True" w438 {
                    tunnel: [z_StateMachineVorlage."590" ("States") z_StateMachineVorlage."511" ("States")] -> w437
                    frame False {
                      # "We've finished!"
                    }
                    frame True {
                      # "Capture next channel"
                    }
                  }
                }
                frame True {
                  # "Go to next z"
                }
              }
              n228 = Bundle By Name(cluster=w427, "bookmark #"=1 ("Z-step")) -> (w426:T1)
            }
            frame True {
              # "Go to next bookmark"
            }
          }
          n229 = Bundle By Name(cluster=w421, "t frame"=0 ("Z-step")) -> (w422:T1)
        }
        frame True {
          # "Capture next t-frame"
        }
      }
    }
    frame "Z-C-T-B" {
      # "Check C"
      n230 = Unbundle By Name(w451) -> ("Z-current"=w454:i32)
      n231 = Unbundle By Name(w451) -> ("Total z steps"=w453:i32)
      n232 = Less?(x=w454, y=w453) -> (x < y?=w452:bool)
      n233 = case shown="False" w452 {
        tunnel: w451 -> [w458 w484]
        tunnel: [w459 z_StateMachineVorlage."513" ("States")] -> w450
        tunnel: [w455 w484] -> w449
        frame False {
          # "Set z-step to 0. Check C"
          n234 = Unbundle By Name(w458) -> ("Total channels"=w462:i32)
          n235 = Unbundle By Name(w458) -> ("Channel"=w461:i32)
          n236 = Less?(x=w461, y=w462) -> (x < y?=w460:bool)
          n237 = case shown="False" w460 {
            tunnel: [w467 z_StateMachineVorlage."511" ("States")] -> w459
            tunnel: w458 -> [w466 w482]
            tunnel: [w463 w482] -> w456
            frame False {
              # "Set C to 0. Check T"
              n238 = Unbundle By Name(w466) -> ("total t frames"=w469:i32)
              n239 = Unbundle By Name(w466) -> ("t frame"=w470:i32)
              n240 = Less?(x=w470, y=w469) -> (x < y?=w468:bool)
              n241 = case shown="False" w468 {
                tunnel: w466 -> [w473 w480]
                tunnel: [w474 z_StateMachineVorlage."512" ("States")] -> w467
                tunnel: [w471 w480] -> w464
                frame False {
                  # "Set T to 0. Check B"
                  n242 = Unbundle By Name(w473) -> ("bookmark #"=w476:i32)
                  n243 = Unbundle By Name(w473) -> ("Total bookmarks"=w477:i32)
                  n244 = Bundle By Name(cluster=w473, "t frame"=1 ("Z-step")) -> (w471:T1)
                  n245 = Less?(x=w476, y=w477) -> (x < y?=w475:bool)
                  n246 = case shown="True" w475 {
                    tunnel: [z_StateMachineVorlage."590" ("States") z_StateMachineVorlage."514" ("States")] -> w474
                    frame False {
                      # "We've finished!"
                    }
                    frame True {
                      # "Go to next bookmark"
                    }
                  }
                }
                frame True {
                  # "Go to next T"
                }
              }
              n247 = Bundle By Name(cluster=w464, "Channel"=1 ("Z-step")) -> (w463:T1)
            }
            frame True {
              # "Capture next channel"
            }
          }
          n248 = Bundle By Name(cluster=w456, "Z-current"=0 ("Z-step")) -> (w455:T1)
        }
        frame True {
          # "Go to next z"
        }
      }
    }
    frame "Z-C-B-T" {
      # "Check C"
      n249 = Unbundle By Name(w488) -> ("Z-current"=w491:i32)
      n250 = Unbundle By Name(w488) -> ("Total z steps"=w490:i32)
      n251 = Less?(x=w491, y=w490) -> (x < y?=w489:bool)
      n252 = case shown="False" w489 {
        tunnel: w488 -> [w495 w521]
        tunnel: [w496 z_StateMachineVorlage."513" ("States")] -> w487
        tunnel: [w492 w521] -> w486
        frame False {
          # "Set z-step to 0. Check C"
          n253 = Unbundle By Name(w495) -> ("Total channels"=w499:i32)
          n254 = Unbundle By Name(w495) -> ("Channel"=w498:i32)
          n255 = Less?(x=w498, y=w499) -> (x < y?=w497:bool)
          n256 = case shown="False" w497 {
            tunnel: [w504 z_StateMachineVorlage."511" ("States")] -> w496
            tunnel: w495 -> [w503 w519]
            tunnel: [w500 w519] -> w493
            frame False {
              # "Set C to 0. Check B"
              n257 = Unbundle By Name(w503) -> ("bookmark #"=w507:i32)
              n258 = Unbundle By Name(w503) -> ("Total bookmarks"=w506:i32)
              n259 = Less?(x=w507, y=w506) -> (x < y?=w505:bool)
              n260 = case shown="False" w505 {
                tunnel: w503 -> [w510 w517]
                tunnel: [w511 z_StateMachineVorlage."514" ("States")] -> w504
                tunnel: [w508 w517] -> w501
                frame False {
                  # "Set B to 0. Check T"
                  n261 = Unbundle By Name(w510) -> ("total t frames"=w514:i32)
                  n262 = Unbundle By Name(w510) -> ("t frame"=w513:i32)
                  n263 = Bundle By Name(cluster=w510, "bookmark #"=1 ("Z-step")) -> (w508:T1)
                  n264 = Less?(x=w513, y=w514) -> (x < y?=w512:bool)
                  n265 = case shown="True" w512 {
                    tunnel: [z_StateMachineVorlage."590" ("States") z_StateMachineVorlage."512" ("States")] -> w511
                    frame False {
                      # "We've finished!"
                    }
                    frame True {
                      # "Go to next t-frame"
                    }
                  }
                }
                frame True {
                  # "Go to next B"
                }
              }
              n266 = Bundle By Name(cluster=w501, "Channel"=1 ("Z-step")) -> (w500:T1)
            }
            frame True {
              # "Capture next channel"
            }
          }
          n267 = Bundle By Name(cluster=w493, "Z-current"=0 ("Z-step")) -> (w492:T1)
        }
        frame True {
          # "Go to next z"
        }
      }
    }
    frame "Z-T-C-B" {
      # "Check C"
      n268 = Unbundle By Name(w525) -> ("Z-current"=w528:i32)
      n269 = Unbundle By Name(w525) -> ("Total z steps"=w527:i32)
      n270 = Less?(x=w528, y=w527) -> (x < y?=w526:bool)
      n271 = case shown="False" w526 {
        tunnel: w525 -> [w532 w558]
        tunnel: [w533 z_StateMachineVorlage."513" ("States")] -> w524
        tunnel: [w529 w558] -> w523
        frame False {
          # "Set z-step to 0. Check C"
          n272 = Unbundle By Name(w532) -> ("total t frames"=w536:i32)
          n273 = Unbundle By Name(w532) -> ("t frame"=w535:i32)
          n274 = Less?(x=w535, y=w536) -> (x < y?=w534:bool)
          n275 = case shown="False" w534 {
            tunnel: [w541 z_StateMachineVorlage."512" ("States")] -> w533
            tunnel: w532 -> [w540 w556]
            tunnel: [w537 w556] -> w530
            frame False {
              # "Set T to 0. Check C"
              n276 = Unbundle By Name(w540) -> ("Total channels"=w543:i32)
              n277 = Unbundle By Name(w540) -> ("Channel"=w544:i32)
              n278 = Less?(x=w544, y=w543) -> (x < y?=w542:bool)
              n279 = case shown="False" w542 {
                tunnel: w540 -> [w547 w554]
                tunnel: [w548 z_StateMachineVorlage."511" ("States")] -> w541
                tunnel: [w545 w554] -> w538
                frame False {
                  # "Set C to 0. Check B"
                  n280 = Unbundle By Name(w547) -> ("bookmark #"=w550:i32)
                  n281 = Unbundle By Name(w547) -> ("Total bookmarks"=w551:i32)
                  n282 = Bundle By Name(cluster=w547, "Channel"=1 ("Z-step")) -> (w545:T1)
                  n283 = Less?(x=w550, y=w551) -> (x < y?=w549:bool)
                  n284 = case shown="True" w549 {
                    tunnel: [z_StateMachineVorlage."590" ("States") z_StateMachineVorlage."514" ("States")] -> w548
                    frame False {
                      # "We've finished!"
                    }
                    frame True {
                      # "Go to next bookmark"
                    }
                  }
                }
                frame True {
                  # "Capture next C"
                }
              }
              n285 = Bundle By Name(cluster=w538, "t frame"=1 ("Z-step")) -> (w537:T1)
            }
            frame True {
              # "Next t-frame"
            }
          }
          n286 = Bundle By Name(cluster=w530, "Z-current"=0 ("Z-step")) -> (w529:T1)
        }
        frame True {
          # "Go to next z"
        }
      }
    }
    frame "Z-T-B-C" {
      # "Check C"
      n287 = Unbundle By Name(w562) -> ("Z-current"=w565:i32)
      n288 = Unbundle By Name(w562) -> ("Total z steps"=w564:i32)
      n289 = Less?(x=w565, y=w564) -> (x < y?=w563:bool)
      n290 = case shown="False" w563 {
        tunnel: w562 -> [w569 w595]
        tunnel: [w570 z_StateMachineVorlage."513" ("States")] -> w561
        tunnel: [w566 w595] -> w560
        frame False {
          # "Set z-step to 0. Check C"
          n291 = Unbundle By Name(w569) -> ("total t frames"=w573:i32)
          n292 = Unbundle By Name(w569) -> ("t frame"=w572:i32)
          n293 = Less?(x=w572, y=w573) -> (x < y?=w571:bool)
          n294 = case shown="False" w571 {
            tunnel: [w578 z_StateMachineVorlage."512" ("States")] -> w570
            tunnel: w569 -> [w577 w593]
            tunnel: [w574 w593] -> w567
            frame False {
              # "Set T to 0. Check C"
              n295 = Unbundle By Name(w577) -> ("bookmark #"=w581:i32)
              n296 = Unbundle By Name(w577) -> ("Total bookmarks"=w580:i32)
              n297 = Less?(x=w581, y=w580) -> (x < y?=w579:bool)
              n298 = case shown="False" w579 {
                tunnel: w577 -> [w584 w591]
                tunnel: [w585 z_StateMachineVorlage."514" ("States")] -> w578
                tunnel: [w582 w591] -> w575
                frame False {
                  # "Set B to 0. Check C"
                  n299 = Unbundle By Name(w584) -> ("Total channels"=w588:i32)
                  n300 = Unbundle By Name(w584) -> ("Channel"=w587:i32)
                  n301 = Bundle By Name(cluster=w584, "bookmark #"=1 ("Z-step")) -> (w582:T1)
                  n302 = Less?(x=w587, y=w588) -> (x < y?=w586:bool)
                  n303 = case shown="True" w586 {
                    tunnel: [z_StateMachineVorlage."590" ("States") z_StateMachineVorlage."511" ("States")] -> w585
                    frame False {
                      # "We've finished!"
                    }
                    frame True {
                      # "Capture next channel"
                    }
                  }
                }
                frame True {
                  # "Go to next bookmark"
                }
              }
              n304 = Bundle By Name(cluster=w575, "t frame"=1 ("Z-step")) -> (w574:T1)
            }
            frame True {
              # "Next t-frame"
            }
          }
          n305 = Bundle By Name(cluster=w567, "Z-current"=0 ("Z-step")) -> (w566:T1)
        }
        frame True {
          # "Go to next z"
        }
      }
    }
    frame "Z-B-C-T" {
      # "Check C"
      n306 = Unbundle By Name(w599) -> ("Z-current"=w602:i32)
      n307 = Unbundle By Name(w599) -> ("Total z steps"=w601:i32)
      n308 = Less?(x=w602, y=w601) -> (x < y?=w600:bool)
      n309 = case shown="False" w600 {
        tunnel: w599 -> [w606 w632]
        tunnel: [w607 z_StateMachineVorlage."513" ("States")] -> w598
        tunnel: [w603 w632] -> w597
        frame False {
          # "Set z-step to 0. Check C"
          n310 = Unbundle By Name(w606) -> ("bookmark #"=w609:i32)
          n311 = Unbundle By Name(w606) -> ("Total bookmarks"=w610:i32)
          n312 = Less?(x=w609, y=w610) -> (x < y?=w608:bool)
          n313 = case shown="False" w608 {
            tunnel: [w615 z_StateMachineVorlage."513" ("States")] -> w607
            tunnel: w606 -> [w614 w630]
            tunnel: [w611 w630] -> w604
            frame False {
              # "Set B to 0. Check C"
              n314 = Unbundle By Name(w614) -> ("Total channels"=w617:i32)
              n315 = Unbundle By Name(w614) -> ("Channel"=w618:i32)
              n316 = Less?(x=w618, y=w617) -> (x < y?=w616:bool)
              n317 = case shown="False" w616 {
                tunnel: w614 -> [w621 w628]
                tunnel: [w622 z_StateMachineVorlage."511" ("States")] -> w615
                tunnel: [w619 w628] -> w612
                frame False {
                  # "Set C to 0. Check T"
                  n318 = Unbundle By Name(w621) -> ("total t frames"=w625:i32)
                  n319 = Unbundle By Name(w621) -> ("t frame"=w624:i32)
                  n320 = Bundle By Name(cluster=w621, "Channel"=1 ("Z-step")) -> (w619:T1)
                  n321 = Less?(x=w624, y=w625) -> (x < y?=w623:bool)
                  n322 = case shown="True" w623 {
                    tunnel: [z_StateMachineVorlage."590" ("States") z_StateMachineVorlage."512" ("States")] -> w622
                    frame False {
                      # "We've finished!"
                    }
                    frame True {
                      # "Go to next T"
                    }
                  }
                }
                frame True {
                  # "Capture next channel"
                }
              }
              n323 = Bundle By Name(cluster=w612, "bookmark #"=1 ("Z-step")) -> (w611:T1)
            }
            frame True {
              # "Go to next bookmark"
            }
          }
          n324 = Bundle By Name(cluster=w604, "Z-current"=0 ("Z-step")) -> (w603:T1)
        }
        frame True {
          # "Go to next z"
        }
      }
    }
    frame "Z-B-T-C" {
      # "Check C"
      n325 = Unbundle By Name(w636) -> ("Z-current"=w639:i32)
      n326 = Unbundle By Name(w636) -> ("Total z steps"=w638:i32)
      n327 = Less?(x=w639, y=w638) -> (x < y?=w637:bool)
      n328 = case shown="False" w637 {
        tunnel: w636 -> [w643 w669]
        tunnel: [w644 z_StateMachineVorlage."513" ("States")] -> w635
        tunnel: [w640 w669] -> w634
        frame False {
          # "Set z-step to 0. Check C"
          n329 = Unbundle By Name(w643) -> ("bookmark #"=w646:i32)
          n330 = Unbundle By Name(w643) -> ("Total bookmarks"=w647:i32)
          n331 = Less?(x=w646, y=w647) -> (x < y?=w645:bool)
          n332 = case shown="False" w645 {
            tunnel: [w652 z_StateMachineVorlage."513" ("States")] -> w644
            tunnel: w643 -> [w651 w667]
            tunnel: [w648 w667] -> w641
            frame False {
              # "Set B to 0. Check T"
              n333 = Unbundle By Name(w651) -> ("total t frames"=w654:i32)
              n334 = Unbundle By Name(w651) -> ("t frame"=w655:i32)
              n335 = Less?(x=w655, y=w654) -> (x < y?=w653:bool)
              n336 = case shown="False" w653 {
                tunnel: w651 -> [w658 w665]
                tunnel: [w659 z_StateMachineVorlage."512" ("States")] -> w652
                tunnel: [w656 w665] -> w649
                frame False {
                  # "Set T to 0. Check C"
                  n337 = Unbundle By Name(w658) -> ("Total channels"=w662:i32)
                  n338 = Unbundle By Name(w658) -> ("Channel"=w661:i32)
                  n339 = Bundle By Name(cluster=w658, "t frame"=1 ("Z-step")) -> (w656:T1)
                  n340 = Less?(x=w661, y=w662) -> (x < y?=w660:bool)
                  n341 = case shown="True" w660 {
                    tunnel: [z_StateMachineVorlage."590" ("States") z_StateMachineVorlage."511" ("States")] -> w659
                    frame False {
                      # "We've finished!"
                    }
                    frame True {
                      # "Capture next channel"
                    }
                  }
                }
                frame True {
                  # "Go to next t-frame"
                }
              }
              n342 = Bundle By Name(cluster=w649, "bookmark #"=1 ("Z-step")) -> (w648:T1)
            }
            frame True {
              # "Go to next bookmark"
            }
          }
          n343 = Bundle By Name(cluster=w641, "Z-current"=0 ("Z-step")) -> (w640:T1)
        }
        frame True {
          # "Go to next z"
        }
      }
    }
    frame "B-C-T-Z" {
      # "Check B"
      n344 = Unbundle By Name(w673) -> ("bookmark #"=w676:i32)
      n345 = Unbundle By Name(w673) -> ("Total bookmarks"=w675:i32)
      n346 = Less?(x=w676, y=w675) -> (x < y?=w674:bool)
      n347 = case shown="False" w674 {
        tunnel: w673 -> [w680 w706]
        tunnel: [w681 z_StateMachineVorlage."514" ("States")] -> w672
        tunnel: [w678 w706] -> w671
        frame False {
          # "Set bookmark to 0. Check C"
          n348 = Unbundle By Name(w680) -> ("Total channels"=w684:i32)
          n349 = Unbundle By Name(w680) -> ("Channel"=w683:i32)
          n350 = Less?(x=w683, y=w684) -> (x < y?=w682:bool)
          n351 = case shown="False" w682 {
            tunnel: [w689 z_StateMachineVorlage."511" ("States")] -> w681
            tunnel: w680 -> [w688 w704]
            tunnel: [w685 w704] -> w679
            frame False {
              # "Set C to 0. Check T"
              n352 = Unbundle By Name(w688) -> ("total t frames"=w691:i32)
              n353 = Unbundle By Name(w688) -> ("t frame"=w692:i32)
              n354 = Less?(x=w692, y=w691) -> (x < y?=w690:bool)
              n355 = case shown="False" w690 {
                tunnel: w688 -> [w695 w702]
                tunnel: [w696 z_StateMachineVorlage."512" ("States")] -> w689
                tunnel: [w693 w702] -> w686
                frame False {
                  # "Set T to 0. Check Z"
                  n356 = Unbundle By Name(w695) -> ("Z-current"=w698:i32)
                  n357 = Unbundle By Name(w695) -> ("Total z steps"=w699:i32)
                  n358 = Bundle By Name(cluster=w695, "t frame"=1 ("Z-step")) -> (w693:T1)
                  n359 = Less?(x=w698, y=w699) -> (x < y?=w697:bool)
                  n360 = case shown="True" w697 {
                    tunnel: [z_StateMachineVorlage."590" ("States") z_StateMachineVorlage."513" ("States")] -> w696
                    frame False {
                      # "We've finished!"
                    }
                    frame True {
                      # "Go to next Z"
                    }
                  }
                }
                frame True {
                  # "Go to next t-frame"
                }
              }
              n361 = Bundle By Name(cluster=w686, "Channel"=1 ("Z-step")) -> (w685:T1)
            }
            frame True {
              # "Capture next channel"
            }
          }
          n362 = Bundle By Name(cluster=w679, "bookmark #"=0 ("Z-step")) -> (w678:T1)
        }
        frame True {
          # "Go to next bookmark"
        }
      }
    }
    frame "B-C-Z-T" {
      # "Check B"
      n363 = Unbundle By Name(w710) -> ("bookmark #"=w713:i32)
      n364 = Unbundle By Name(w710) -> ("Total bookmarks"=w712:i32)
      n365 = Less?(x=w713, y=w712) -> (x < y?=w711:bool)
      n366 = case shown="False" w711 {
        tunnel: w710 -> [w717 w743]
        tunnel: [w718 z_StateMachineVorlage."514" ("States")] -> w709
        tunnel: [w714 w743] -> w708
        frame False {
          # "Set bookmark to 0. Check C"
          n367 = Unbundle By Name(w717) -> ("Total channels"=w721:i32)
          n368 = Unbundle By Name(w717) -> ("Channel"=w720:i32)
          n369 = Less?(x=w720, y=w721) -> (x < y?=w719:bool)
          n370 = case shown="False" w719 {
            tunnel: [w726 z_StateMachineVorlage."511" ("States")] -> w718
            tunnel: w717 -> [w725 w741]
            tunnel: [w722 w741] -> w715
            frame False {
              # "Set C to 0. Check Z"
              n371 = Unbundle By Name(w725) -> ("Total z steps"=w728:i32)
              n372 = Unbundle By Name(w725) -> ("Z-current"=w729:i32)
              n373 = Less?(x=w729, y=w728) -> (x < y?=w727:bool)
              n374 = case shown="False" w727 {
                tunnel: w725 -> [w732 w739]
                tunnel: [w733 z_StateMachineVorlage."513" ("States")] -> w726
                tunnel: [w730 w739] -> w723
                frame False {
                  # "Set Z to 0. Check T"
                  n375 = Unbundle By Name(w732) -> ("total t frames"=w736:i32)
                  n376 = Unbundle By Name(w732) -> ("t frame"=w735:i32)
                  n377 = Bundle By Name(cluster=w732, "Z-current"=1 ("Z-step")) -> (w730:T1)
                  n378 = Less?(x=w735, y=w736) -> (x < y?=w734:bool)
                  n379 = case shown="True" w734 {
                    tunnel: [z_StateMachineVorlage."590" ("States") z_StateMachineVorlage."512" ("States")] -> w733
                    frame False {
                      # "We've finished!"
                    }
                    frame True {
                      # "Go to next T"
                    }
                  }
                }
                frame True {
                  # "Go to next Z"
                }
              }
              n380 = Bundle By Name(cluster=w723, "Channel"=1 ("Z-step")) -> (w722:T1)
            }
            frame True {
              # "Capture next channel"
            }
          }
          n381 = Bundle By Name(cluster=w715, "bookmark #"=0 ("Z-step")) -> (w714:T1)
        }
        frame True {
          # "Go to next bookmark"
        }
      }
    }
    frame "B-Z-C-T" {
      # "Check B"
      n382 = Unbundle By Name(w747) -> ("bookmark #"=w750:i32)
      n383 = Unbundle By Name(w747) -> ("Total bookmarks"=w749:i32)
      n384 = Less?(x=w750, y=w749) -> (x < y?=w748:bool)
      n385 = case shown="False" w748 {
        tunnel: w747 -> [w755 w780]
        tunnel: [w756 z_StateMachineVorlage."514" ("States")] -> w746
        tunnel: [w752 w780] -> w745
        frame False {
          # "Set bookmark to 0. Check Z"
          n386 = Unbundle By Name(w755) -> ("Z-current"=w751:i32)
          n387 = Unbundle By Name(w755) -> ("Total z steps"=w758:i32)
          n388 = Less?(x=w751, y=w758) -> (x < y?=w757:bool)
          n389 = case shown="False" w757 {
            tunnel: [w763 z_StateMachineVorlage."513" ("States")] -> w756
            tunnel: w755 -> [w762 w778]
            tunnel: [w759 w778] -> w753
            frame False {
              # "Set Z to 0. Check C"
              n390 = Unbundle By Name(w762) -> ("Total channels"=w765:i32)
              n391 = Unbundle By Name(w762) -> ("Channel"=w766:i32)
              n392 = Less?(x=w766, y=w765) -> (x < y?=w764:bool)
              n393 = case shown="False" w764 {
                tunnel: w762 -> [w769 w776]
                tunnel: [w770 z_StateMachineVorlage."511" ("States")] -> w763
                tunnel: [w767 w776] -> w760
                frame False {
                  # "Set C to 0. Check T"
                  n394 = Unbundle By Name(w769) -> ("total t frames"=w773:i32)
                  n395 = Unbundle By Name(w769) -> ("t frame"=w772:i32)
                  n396 = Bundle By Name(cluster=w769, "Channel"=1 ("Z-step")) -> (w767:T1)
                  n397 = Less?(x=w772, y=w773) -> (x < y?=w771:bool)
                  n398 = case shown="True" w771 {
                    tunnel: [z_StateMachineVorlage."590" ("States") z_StateMachineVorlage."512" ("States")] -> w770
                    frame False {
                      # "We've finished!"
                    }
                    frame True {
                      # "Go to next T"
                    }
                  }
                }
                frame True {
                  # "Capture next channel"
                }
              }
              n399 = Bundle By Name(cluster=w760, "Z-current"=1 ("Z-step")) -> (w759:T1)
            }
            frame True {
              # "Go to next Z"
            }
          }
          n400 = Bundle By Name(cluster=w753, "bookmark #"=0 ("Z-step")) -> (w752:T1)
        }
        frame True {
          # "Go to next bookmark"
        }
      }
    }
    frame "B-Z-T-C" {
      # "Check B"
      n401 = Unbundle By Name(w784) -> ("bookmark #"=w787:i32)
      n402 = Unbundle By Name(w784) -> ("Total bookmarks"=w786:i32)
      n403 = Less?(x=w787, y=w786) -> (x < y?=w785:bool)
      n404 = case shown="False" w785 {
        tunnel: w784 -> [w791 w817]
        tunnel: [w792 z_StateMachineVorlage."514" ("States")] -> w783
        tunnel: [w788 w817] -> w782
        frame False {
          # "Set bookmark to 0. Check Z"
          n405 = Unbundle By Name(w791) -> ("Z-current"=w794:i32)
          n406 = Unbundle By Name(w791) -> ("Total z steps"=w795:i32)
          n407 = Less?(x=w794, y=w795) -> (x < y?=w793:bool)
          n408 = case shown="False" w793 {
            tunnel: [w800 z_StateMachineVorlage."513" ("States")] -> w792
            tunnel: w791 -> [w799 w815]
            tunnel: [w796 w815] -> w789
            frame False {
              # "Set Z to 0. Check T"
              n409 = Unbundle By Name(w799) -> ("total t frames"=w802:i32)
              n410 = Unbundle By Name(w799) -> ("t frame"=w803:i32)
              n411 = Less?(x=w803, y=w802) -> (x < y?=w801:bool)
              n412 = case shown="False" w801 {
                tunnel: w799 -> [w806 w813]
                tunnel: [w807 z_StateMachineVorlage."512" ("States")] -> w800
                tunnel: [w804 w813] -> w797
                frame False {
                  # "Set T to 0. Check C"
                  n413 = Unbundle By Name(w806) -> ("Total channels"=w810:i32)
                  n414 = Unbundle By Name(w806) -> ("Channel"=w809:i32)
                  n415 = Bundle By Name(cluster=w806, "t frame"=1 ("Z-step")) -> (w804:T1)
                  n416 = Less?(x=w809, y=w810) -> (x < y?=w808:bool)
                  n417 = case shown="True" w808 {
                    tunnel: [z_StateMachineVorlage."590" ("States") z_StateMachineVorlage."511" ("States")] -> w807
                    frame False {
                      # "We've finished!"
                    }
                    frame True {
                      # "Capture next channel"
                    }
                  }
                }
                frame True {
                  # "Go to next t-frame"
                }
              }
              n418 = Bundle By Name(cluster=w797, "Z-current"=1 ("Z-step")) -> (w796:T1)
            }
            frame True {
              # "Go to next Z step"
            }
          }
          n419 = Bundle By Name(cluster=w789, "bookmark #"=0 ("Z-step")) -> (w788:T1)
        }
        frame True {
          # "Go to next bookmark"
        }
      }
    }
    frame "B-T-C-Z" {
      # "Check B"
      n420 = Unbundle By Name(w821) -> ("bookmark #"=w824:i32)
      n421 = Unbundle By Name(w821) -> ("Total bookmarks"=w823:i32)
      n422 = Less?(x=w824, y=w823) -> (x < y?=w822:bool)
      n423 = case shown="False" w822 {
        tunnel: w821 -> [w826 w854]
        tunnel: [w825 z_StateMachineVorlage."514" ("States")] -> w820
        tunnel: [w829 w854] -> w819
        frame False {
          # "Set bookmark to 0. Check T"
          n424 = Unbundle By Name(w826) -> ("t frame"=w831:i32)
          n425 = Unbundle By Name(w826) -> ("total t frames"=w832:i32)
          n426 = Less?(x=w831, y=w832) -> (x < y?=w827:bool)
          n427 = case shown="False" w827 {
            tunnel: [w837 z_StateMachineVorlage."512" ("States")] -> w825
            tunnel: w826 -> [w836 w852]
            tunnel: [w833 w852] -> w828
            frame False {
              # "Set T to 0. Check C"
              n428 = Unbundle By Name(w836) -> ("Total channels"=w839:i32)
              n429 = Unbundle By Name(w836) -> ("Channel"=w840:i32)
              n430 = Less?(x=w840, y=w839) -> (x < y?=w838:bool)
              n431 = case shown="False" w838 {
                tunnel: w836 -> [w843 w850]
                tunnel: [w844 z_StateMachineVorlage."511" ("States")] -> w837
                tunnel: [w841 w850] -> w834
                frame False {
                  # "Set C to 0. Check Z"
                  n432 = Unbundle By Name(w843) -> ("Z-current"=w846:i32)
                  n433 = Unbundle By Name(w843) -> ("Total z steps"=w847:i32)
                  n434 = Bundle By Name(cluster=w843, "Channel"=1 ("Z-step")) -> (w841:T1)
                  n435 = Less?(x=w846, y=w847) -> (x < y?=w845:bool)
                  n436 = case shown="True" w845 {
                    tunnel: [z_StateMachineVorlage."590" ("States") z_StateMachineVorlage."513" ("States")] -> w844
                    frame False {
                      # "We've finished!"
                    }
                    frame True {
                      # "Go to next Z"
                    }
                  }
                }
                frame True {
                  # "Capture next channel"
                }
              }
              n437 = Bundle By Name(cluster=w834, "t frame"=1 ("Z-step")) -> (w833:T1)
            }
            frame True {
              # "Go to next t-frame"
            }
          }
          n438 = Bundle By Name(cluster=w828, "bookmark #"=0 ("Z-step")) -> (w829:T1)
        }
        frame True {
          # "Go to next bookmark"
        }
      }
    }
    frame "B-T-Z-C" {
      # "Check B"
      n439 = Unbundle By Name(w858) -> ("bookmark #"=w861:i32)
      n440 = Unbundle By Name(w858) -> ("Total bookmarks"=w860:i32)
      n441 = Less?(x=w861, y=w860) -> (x < y?=w859:bool)
      n442 = case shown="False" w859 {
        tunnel: w858 -> [w863 w891]
        tunnel: [w862 z_StateMachineVorlage."514" ("States")] -> w857
        tunnel: [w866 w891] -> w856
        frame False {
          # "Set bookmark to 0. Check T"
          n443 = Unbundle By Name(w863) -> ("t frame"=w868:i32)
          n444 = Unbundle By Name(w863) -> ("total t frames"=w869:i32)
          n445 = Less?(x=w868, y=w869) -> (x < y?=w864:bool)
          n446 = case shown="False" w864 {
            tunnel: [w874 z_StateMachineVorlage."512" ("States")] -> w862
            tunnel: w863 -> [w873 w889]
            tunnel: [w870 w889] -> w865
            frame False {
              # "Set T to 0. Check Z"
              n447 = Unbundle By Name(w873) -> ("Z-current"=w877:i32)
              n448 = Unbundle By Name(w873) -> ("Total z steps"=w876:i32)
              n449 = Less?(x=w877, y=w876) -> (x < y?=w875:bool)
              n450 = case shown="False" w875 {
                tunnel: w873 -> [w880 w887]
                tunnel: [w881 z_StateMachineVorlage."513" ("States")] -> w874
                tunnel: [w878 w887] -> w871
                frame False {
                  # "Set Z to 0. Check C"
                  n451 = Unbundle By Name(w880) -> ("Total channels"=w884:i32)
                  n452 = Unbundle By Name(w880) -> ("Channel"=w883:i32)
                  n453 = Bundle By Name(cluster=w880, "Z-current"=1 ("Z-step")) -> (w878:T1)
                  n454 = Less?(x=w883, y=w884) -> (x < y?=w882:bool)
                  n455 = case shown="True" w882 {
                    tunnel: [z_StateMachineVorlage."590" ("States") z_StateMachineVorlage."511" ("States")] -> w881
                    frame False {
                      # "We've finished!"
                    }
                    frame True {
                      # "Capture next channel"
                    }
                  }
                }
                frame True {
                  # "Go to next z-step"
                }
              }
              n456 = Bundle By Name(cluster=w871, "t frame"=1 ("Z-step")) -> (w870:T1)
            }
            frame True {
              # "Go to next t-frame"
            }
          }
          n457 = Bundle By Name(cluster=w865, "bookmark #"=0 ("Z-step")) -> (w866:T1)
        }
        frame True {
          # "Go to next bookmark"
        }
      }
    }
  }
  "Next state" <- w3
  "Acquisition cluster out" <- w1
